vi "Enumerate Capture Devices.vi"(8 "error in (no error)":errorcluster) -> (0 "error out":errorcluster, 3 "Devices":map{string, T1}(c390))   [LabVIEW 2020, in "g_ar_toolkit.capture.lvlib"]
uses:
  Stream/Device Enumeration.ctl
  Stream/Stream Parameters.ctl
  g_ar_toolkit.capture.lvlib
  Stream/Stream.lvclass
  g_ar_toolkit.common/g_ar_toolkit.common.lvlib
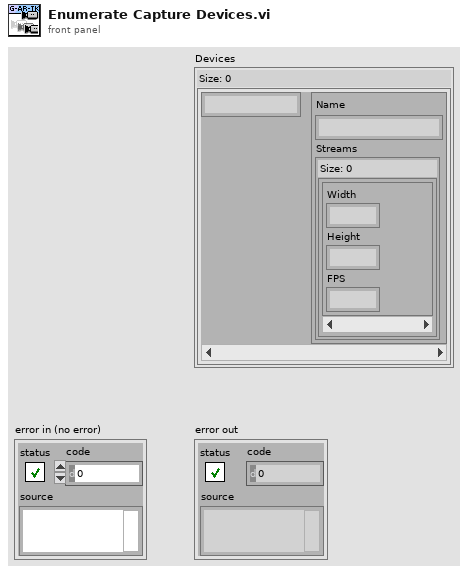
[diagram p1: front panel]
types:
  T1 = typedef "g_ar_toolkit.capture.lvlib/Stream.lvclass/Device Enumeration.ctl" = cluster{"Name":string, "Streams":set{T2}}
  T2 = typedef "g_ar_toolkit.capture.lvlib/Stream.lvclass/Stream Parameters.ctl" = cluster{"Width":u16, "Height":u16, "FPS":u8}
  T3 = cluster{"id":string, "name":string, cluster{"width":u32, "height":u32, "fps_n":u32, "fps_d":u32}[]}[]
  T4 = cluster{"width":u32, "height":u32, "fps_n":u32, "fps_d":u32}[]
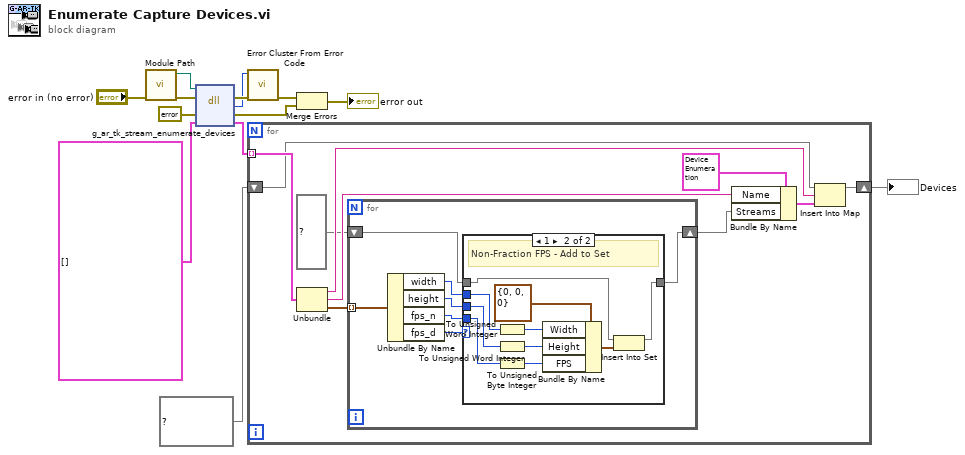
[diagram p0: block diagram]
diagram:
  n1 = call "Module Path.vi"("error in (no error)"="error in (no error)") -> ("error out"=w2:errorcluster, "Path"=w1:path)  [unwired: 9 in]
  n2 = dll-call lib="?" fn="g_ar_tk_stream_enumerate_devices" ("g_ar_toolkit.*.*:g_ar_tk_capture_context_enumerate")(path in=w1, error in=w2, "error_cluster"=errorcluster {"status"=FALSE, "code"=0, "source"=""} ("error constant"), "device_list"=T3 []) -> (error out=w12:errorcluster, "MgErr"=w8:i32, "error_cluster"=w9:errorcluster, "device_list"=w6:T3)  [unwired: 1 in, 1 out]
  n3 = call <vilib>:"Error Cluster From Error Code.vi"("error in (no error)"=w12, "error code (0)"=w8) -> ("error out"=w11:errorcluster)  [unwired: 7 in]
  n4 = for {
    tunnel: w6 -> [w23] mode=indexing
    shift-right: [w19] -> w13
    shift-left: map{string, T1} {} ("Size: 0") -> [w18]
    n5 = Unbundle(w23) -> ("id"=w17:string, "name"=w21:string, w22:T4)
    n6 = for {
      tunnel: w22 -> [w30] mode=indexing
      shift-right: [w26] -> w15
      shift-left: set{T2} {} ("Size: 0") -> [w25]
      n7 = Unbundle By Name(w30) -> ("width"=w27:u32, "height"=w28:u32, "fps_n"=w29:u32, "fps_d"=w24:u32)
      n8 = case shown="1" w24 {
        tunnel: w29 -> [_ w41]
        tunnel: w28 -> [_ w40]
        tunnel: w27 -> [_ w39]
        tunnel: [w31 w38] -> w26
        tunnel: w25 -> [w31 w37]
        frame Default {
          # "Fractional FPS - Skip"
        }
        frame 1 {
          # "Non-Fraction FPS - Add to Set"
          n9 = To Unsigned Word Integer(number=w39) -> (unsigned 16bit integer=w35:u16)
          n10 = To Unsigned Word Integer(number=w40) -> (unsigned 16bit integer=w34:u16)
          n11 = To Unsigned Byte Integer(number=w41) -> (unsigned 8bit integer=w33:u8)
          n12 = Bundle By Name(cluster=T2 {"Width"=0, "Height"=0, "FPS"=0} ("Parameters"), "Width"=w35, "Height"=w34, "FPS"=w33) -> (w32:T2)
          n13 = Insert Into Set(10:w32, 11:w37) -> (3:w38:set{T2})  [unwired: 1 out]
        }
      }
    }
    n14 = Bundle By Name(cluster=T1 {"Name"="", "Streams"={}} ("Device Enumeration"), "Name"=w21, "Streams"=w15) -> (w20:T1)
    n15 = Insert Into Map(map in=w18, key=w17, value=w20) -> (map out=w19:map{string, T1})  [unwired: 2 out]
  }
  "Devices" <- w13
  n16 = Merge Errors(w11, w9) -> (→"error out":errorcluster)
